vi "incline.vi"() -> ()   [LabVIEW 2018]
uses:
  MotorController/#include/Global textParse.vi
  <instrlib>/RIGOL DS1000 Series/RIGOL DS1000 Series.lvlib
panel:
  out "Down":bool
  out "Down Measure":dbl
  out "Up Measure":dbl
  out "Up":bool
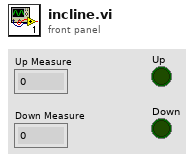
[diagram p1: front panel]
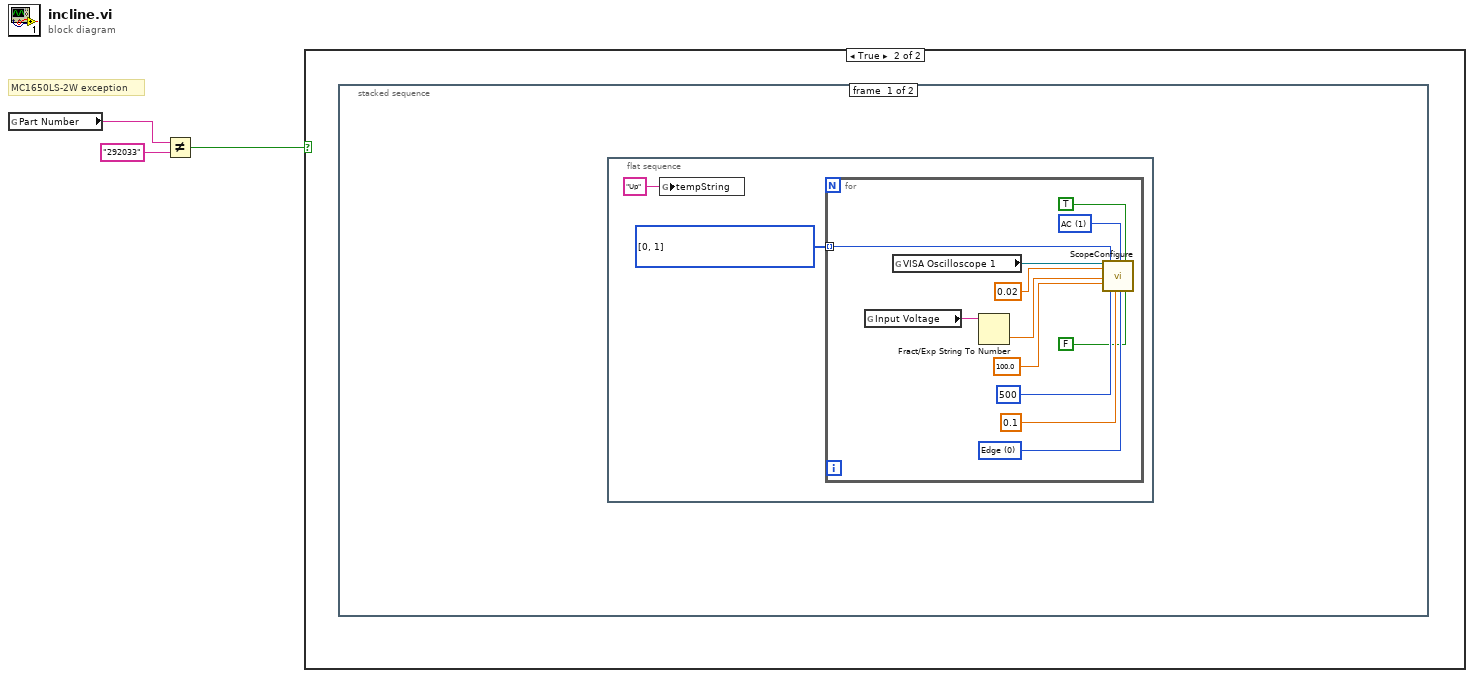
[diagram p0: block diagram]
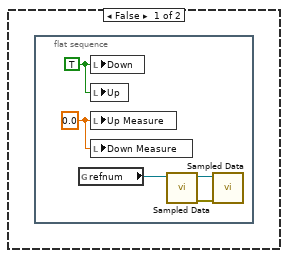
[diagram p2: hidden frame]
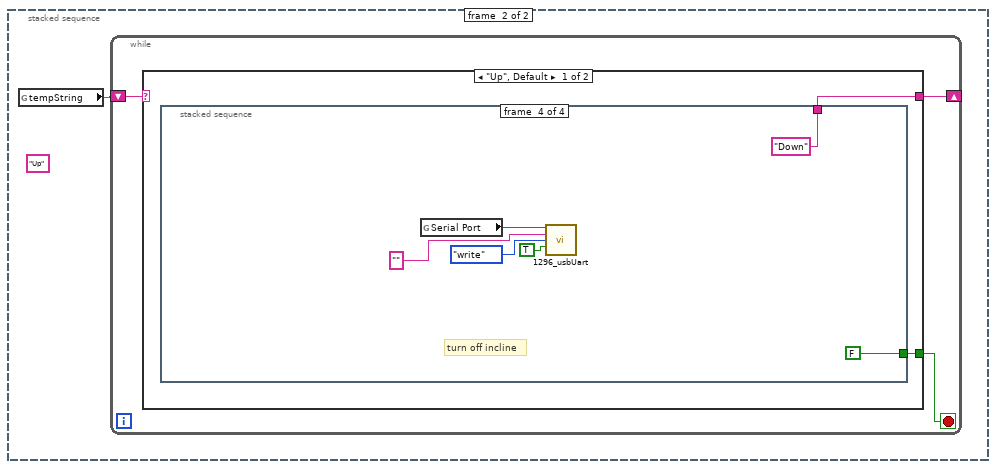
[diagram p3: hidden frame]
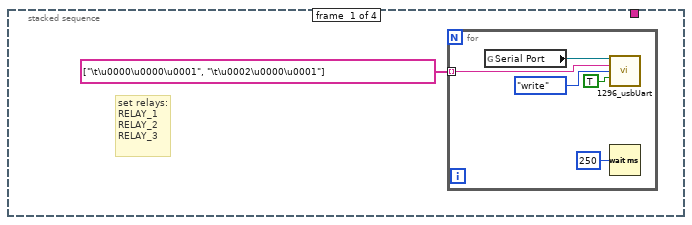
[diagram p4: hidden frame]
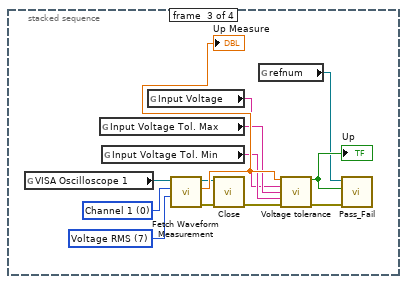
[diagram p6: hidden frame]
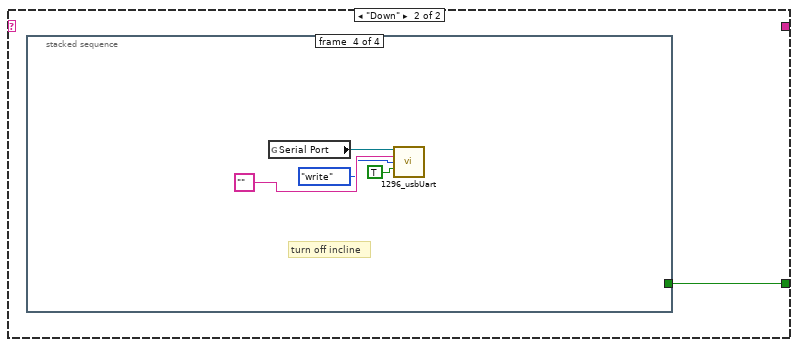
[diagram p7: hidden frame]
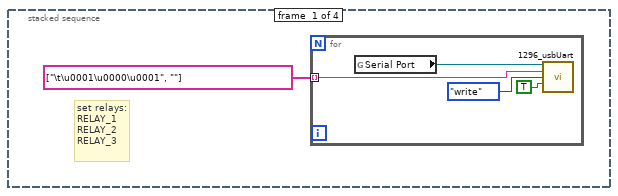
[diagram p8: hidden frame]
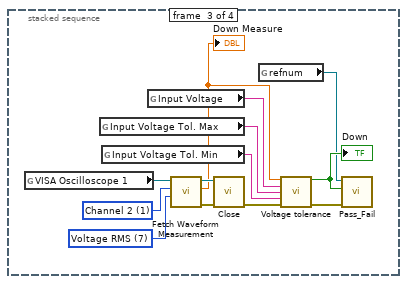
[diagram p10: hidden frame]
diagram:
  # "MC1650LS-2W exception"
  n1 = global read "Global textParse.vi" "Part Number"() -> (w3:string)
  n2 = Not Equal?(x=w3, y="292033") -> (x != y?=w2:bool)
  n3 = case shown="True" w2 {
    frame False {
      n4 = flat-sequence {
        frame #0 {
          w6 = 0.0 ("Up Measure")
          w5 = TRUE ("Up")
          n5 = global read "Global textParse.vi" "refnum"() -> (w4:refnum<file>)
          n6 = local write "Down"(w5) -> ()
          n7 = local write "Up"(w5) -> ()
          n8 = local write "Up Measure"(w6) -> ()
          n9 = local write "Down Measure"(w6) -> ()
          n10 = call "Sampled Data.vi"("refnum in"=w4) -> ("error out"=w7:errorcluster, "refnum out"=w8:refnum<file>)  [unwired: 9 in]
          n11 = call "Sampled Data.vi"("Error In"=w7, "refnum in"=w8) -> ()  [unwired: 8 in, 2 out]
        }
      }
    }
    frame True {
      n12 = stacked-sequence {
        frame #0 {
          n13 = flat-sequence {
            frame #0 {
              w10 = u16[] [0, 1] items=["Channel 1", "Channel 2", "Channel 3", "Channel 4"]
              n14 = global write "Global textParse.vi" "tempString"("Up" ("tempString")) -> ()
              n15 = for {
                tunnel: w10 -> [w11] mode=indexing
                w15 = u16 1 items=["DC", "AC", "Ground"] ("Vertical Coupling (0: DC)")
                w14 = u16 0 items=["Edge", "Pulse", "Video", "Pattern", "Duration"] ("Trigger Type (0: Edge)")
                n16 = global read "Global textParse.vi" "Input Voltage"() -> (w21:string)
                n17 = global read "Global textParse.vi" "VISA Oscilloscope 1"() -> (w22:refnum<visa-resource-name>)
                n18 = Fract/Exp String To Number(string=w21) -> (number=w20:dbl)  [unwired: 3 in, 1 out]
                n19 = call "ScopeConfigure.vi"("VISA resource name"=w22, "scaleTime"=0.02, "triggerVoltage"=w20, "scaleVoltage"=100.0, "Channel (0: Channel 1)"=w11, "Attenuation"=500, "offsetTime"=0.1, "Vertical Coupling (0: DC)"=w15, "Trigger Type (0: Edge)"=w14, "BW Selector"=TRUE, "F Selector"=FALSE) -> ()  [unwired: 7 in, 2 out]
              }
            }
          }
        }
        frame #1 {
          (unwired) "Up"
          n20 = global read "Global textParse.vi" "tempString"() -> (w23:string)
          n21 = while {
            shift-right: [w25] -> _
            shift-left: w23 -> [w26]
            stop <- w24 stop-if-true
            n22 = case shown="\"Up\", Default" w26 {
              tunnel: [w28 _] -> w25
              tunnel: [w27 w54] -> w24
              frame "Up", Default {
                n23 = stacked-sequence {
                  tunnel: [_ _ _ "Down"] -> w28
                  tunnel: [_ _ _ FALSE] -> w27
                  frame #0 {
                    # "set relays:\nRELAY_1\nRELAY_2\nRELAY_3"
                    n24 = for {
                      tunnel: string[] ["\t\u0000\u0000\u0001", "\t\u0002\u0000\u0001"] -> [w31] mode=indexing
                      n25 = global read "Global textParse.vi" "Serial Port"() -> (w34:refnum<visa-resource-name>)
                      n26 = call "1296_usbUart.vi"("VISA resource name"=w34, "command"=w31, "r/w"=enum16{"read", "write"}."write", "resetValues"=TRUE) -> ()  [unwired: 8 in, 4 out]
                      n27 = Wait (ms)(milliseconds to wait=u32 250) -> ()  [unwired: 1 out]
                    }
                  }
                  frame #1 {
                    # "Drive incline"
                  }
                  frame #2 {
                    w38 = u16 7 items=["Voltage Vpp", "Voltage Max", "Voltage Min", "Amplitude", "Voltage TOP", "Voltage Base", "Voltage Average", "Voltage RMS", "Overshoot", "Preshoot", "Frequency", "Rise Time", "Fall Time", "Period", "Positive Width", "Negative Width", "Positive Duty", "Negative Duty"] ("Measurement Function (0: Voltage Vpp)")
                    w37 = u16 0 items=["Channel 1", "Channel 2", "Channel 3", "Channel 4"] ("Source (0: Channel 1)")
                    n28 = global read "Global textParse.vi" "VISA Oscilloscope 1"() -> (w36:refnum<visa-resource-name>)
                    n29 = global read "Global textParse.vi" "Input Voltage Tol. Max"() -> (w42:string)
                    n30 = global read "Global textParse.vi" "Input Voltage Tol. Min"() -> (w43:string)
                    n31 = global read "Global textParse.vi" "Input Voltage"() -> (w41:string)
                    n32 = call <instrlib>:"Fetch Waveform Measurement.vi"("Measurement Function (0: Voltage Vpp)"=w38, "Source (0: Channel 1)"=w37, "VISA resource name"=w36) -> ("error out"=w40:errorcluster, "Measured Value"=w44:dbl, "VISA resource name out"=w39:refnum<visa-resource-name>)  [unwired: 6 in]
                    "Up Measure" <- w44
                    n33 = call <instrlib>:"Close.vi"("error in (no error)"=w40, "VISA resource name"=w39) -> ("error out"=w46:errorcluster)  [unwired: 9 in]
                    n34 = global read "Global textParse.vi" "refnum"() -> (w35:refnum<file>)
                    n35 = call "Voltage tolerance.vi"("Data Sample"=w44, "Spec Output"=w41, "Upper"=w42, "Lower"=w43, "error in (no error)"=w46) -> ("Boolean"=w47:bool, "error out"=w45:errorcluster)  [unwired: 9 in]
                    "Up" <- w47
                    n36 = call "Pass_Fail.vi"("error in (no error)"=w45, "OK"=w47, "Byte Stream File in"=w35) -> ()  [unwired: 7 in, 2 out]
                  }
                  frame #3 {
                    # "turn off incline"
                    n37 = global read "Global textParse.vi" "Serial Port"() -> (w53:refnum<visa-resource-name>)
                    n38 = call "1296_usbUart.vi"("VISA resource name"=w53, "command"="", "r/w"=enum16{"read", "write"}."write", "resetValues"=TRUE) -> ()  [unwired: 8 in, 4 out]
                  }
                }
              }
              frame "Down" {
                n39 = stacked-sequence {
                  tunnel: [_ _ _ _] -> w54
                  frame #0 {
                    # "set relays:\nRELAY_1\nRELAY_2\nRELAY_3"
                    n40 = for {
                      tunnel: string[] ["\t\u0001\u0000\u0001", ""] -> [w56] mode=indexing
                      n41 = global read "Global textParse.vi" "Serial Port"() -> (w59:refnum<visa-resource-name>)
                      n42 = call "1296_usbUart.vi"("VISA resource name"=w59, "command"=w56, "r/w"=enum16{"read", "write"}."write", "resetValues"=TRUE) -> ()  [unwired: 8 in, 4 out]
                    }
                  }
                  frame #1 {
                    # "drive incline"
                  }
                  frame #2 {
                    w65 = u16 7 items=["Voltage Vpp", "Voltage Max", "Voltage Min", "Amplitude", "Voltage TOP", "Voltage Base", "Voltage Average", "Voltage RMS", "Overshoot", "Preshoot", "Frequency", "Rise Time", "Fall Time", "Period", "Positive Width", "Negative Width", "Positive Duty", "Negative Duty"] ("Measurement Function (0: Voltage Vpp)")
                    w64 = u16 1 items=["Channel 1", "Channel 2", "Channel 3", "Channel 4"] ("Source (0: Channel 1)")
                    n43 = global read "Global textParse.vi" "VISA Oscilloscope 1"() -> (w61:refnum<visa-resource-name>)
                    n44 = global read "Global textParse.vi" "Input Voltage Tol. Max"() -> (w69:string)
                    n45 = global read "Global textParse.vi" "Input Voltage Tol. Min"() -> (w70:string)
                    n46 = global read "Global textParse.vi" "Input Voltage"() -> (w68:string)
                    n47 = call <instrlib>:"Fetch Waveform Measurement.vi"("Measurement Function (0: Voltage Vpp)"=w65, "Source (0: Channel 1)"=w64, "VISA resource name"=w61) -> ("error out"=w67:errorcluster, "Measured Value"=w62:dbl, "VISA resource name out"=w66:refnum<visa-resource-name>)  [unwired: 6 in]
                    "Down Measure" <- w62
                    n48 = call <instrlib>:"Close.vi"("error in (no error)"=w67, "VISA resource name"=w66) -> ("error out"=w72:errorcluster)  [unwired: 9 in]
                    n49 = global read "Global textParse.vi" "refnum"() -> (w60:refnum<file>)
                    n50 = call "Voltage tolerance.vi"("Data Sample"=w62, "Spec Output"=w68, "Upper"=w69, "Lower"=w70, "error in (no error)"=w72) -> ("Boolean"=w63:bool, "error out"=w71:errorcluster)  [unwired: 9 in]
                    "Down" <- w63
                    n51 = call "Pass_Fail.vi"("error in (no error)"=w71, "OK"=w63, "Byte Stream File in"=w60) -> ()  [unwired: 7 in, 2 out]
                  }
                  frame #3 {
                    # "turn off incline"
                    n52 = global read "Global textParse.vi" "Serial Port"() -> (w76:refnum<visa-resource-name>)
                    n53 = call "1296_usbUart.vi"("VISA resource name"=w76, "command"="", "r/w"=enum16{"read", "write"}."write", "resetValues"=TRUE) -> ()  [unwired: 8 in, 4 out]
                  }
                }
              }
            }
          }
        }
      }
    }
  }
